vi "adam_init.vi"(10 "Address":i32=3, 11 "COM Port":i32=3) -> (0 "错误输出":errorcluster, 2 "com":refnum<k24>, 3 "modbus":refnum<k24>)   [LabVIEW 2014]
uses:
  ModbusRTU/bin/Debug/Advantech.Adam.dll
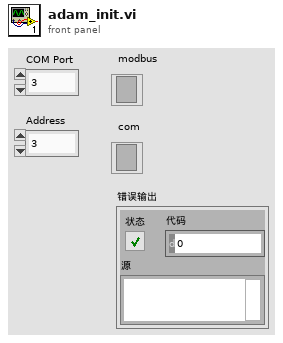
[diagram p1: front panel]
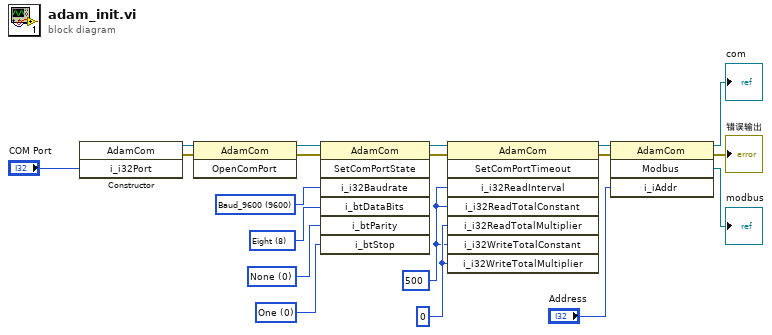
[diagram p0: block diagram]
diagram:
  w12 = 0 ("i_i32ReadTotalMultiplier")
  w11 = 500 ("i_i32ReadInterval")
  w8 = u8 0 items=["One", "OneAndHalf", "Two"] ("i_btStop")
  w7 = u8 0 items=["None", "Odd", "Even", "Mark", "Space"] ("i_btParity")
  w6 = u8 8 items=["Five"=5, "Six"=6, "Seven"=7, "Eight"=8] ("i_btDataBits")
  w5 = 9600 items=["Baud_110"=110, "Baud_300"=300, "Baud_600"=600, "Baud_1200"=1200, "Baud_2400"=2400, "Baud_4800"=4800, "Baud_9600"=9600, "Baud_14400"=14400, "Baud_19200"=19200, "Baud_38400"=38400, "Baud_56000"=56000, "Baud_57600"=57600, "Baud_115200"=115200, "Baud_128000"=128000, "Baud_256000"=256000] ("i_i32Baudrate")
  n1 = constructor class="AdamCom"("i_i32Port"="COM Port") -> (reference out=w1:refnum<k24>, error out=w2:errorcluster)  [unwired: 3 in, 2 out]
  n2 = invoke class="AdamCom" method="OpenComPort"(reference=w1, error in=w2) -> (reference out=w4:refnum<k24>, error out=w3:errorcluster)  [unwired: 1 in, 1 out]
  n3 = invoke class="AdamCom" method="SetComPortState"(reference=w4, error in=w3, "i_i32Baudrate"=w5, "i_btDataBits"=w6, "i_btParity"=w7, "i_btStop"=w8) -> (reference out=w10:refnum<k24>, error out=w9:errorcluster)  [unwired: 1 in, 5 out]
  n4 = invoke class="AdamCom" method="SetComPortTimeout"(reference=w10, error in=w9, "i_i32ReadInterval"=w11, "i_i32ReadTotalConstant"=w11, "i_i32ReadTotalMultiplier"=w12, "i_i32WriteTotalConstant"=w11, "i_i32WriteTotalMultiplier"=w12) -> (reference out=w13:refnum<k24>, error out=w14:errorcluster)  [unwired: 1 in, 6 out]
  n5 = invoke class="AdamCom" method="Modbus"(reference=w13, error in=w14, "i_iAddr"="Address") -> (reference out=→"com":refnum<k24>, error out=→"错误输出":errorcluster, "Modbus"=→"modbus":refnum<k24>)  [unwired: 1 in, 1 out]
